vi "SetDiodeTemp.vi"() -> ()   [LabVIEW 2009]
panel:
  in  "Temp":dbl
  in  "Settling Time (s)":dbl=60.0 caption="Delay Time (s)"
  in  "+e":dbl
  in  "-e":dbl
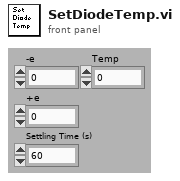
[diagram p1: front panel]
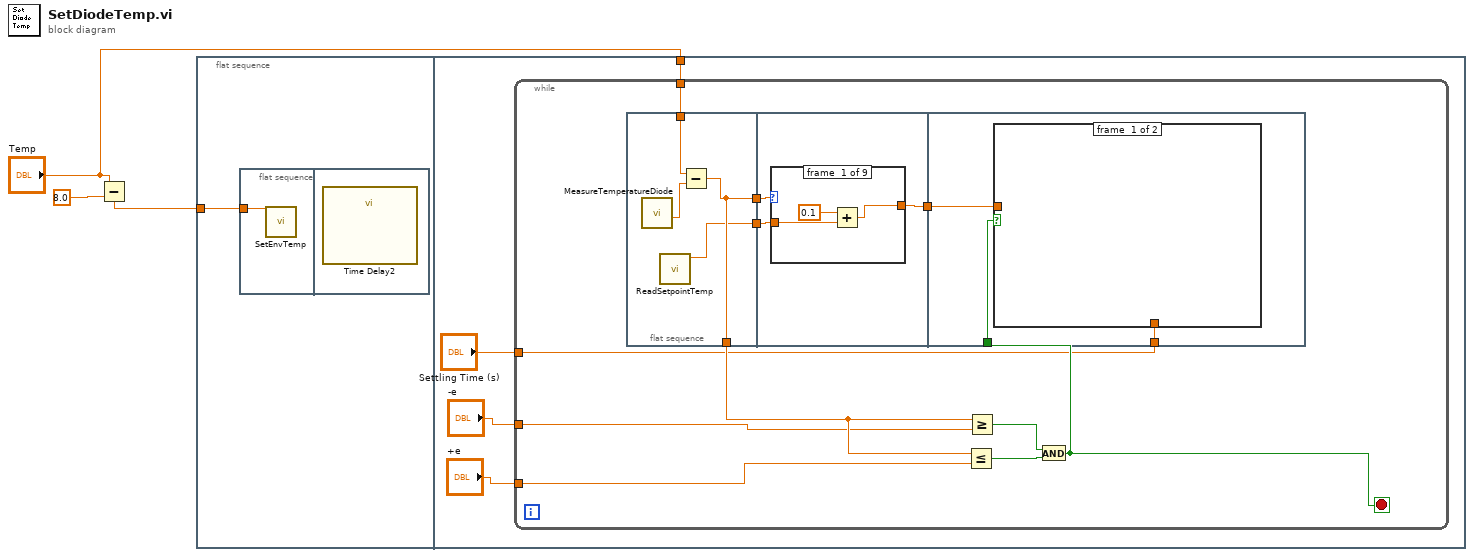
[diagram p0: block diagram]
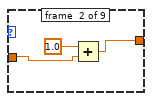
[diagram p2: hidden frame]
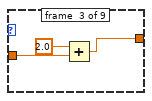
[diagram p3: hidden frame]
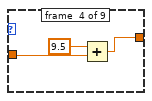
[diagram p4: hidden frame]
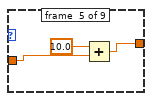
[diagram p5: hidden frame]
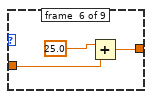
[diagram p6: hidden frame]
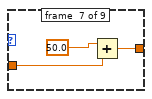
[diagram p7: hidden frame]
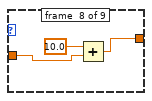
[diagram p8: hidden frame]
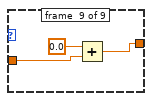
[diagram p9: hidden frame]
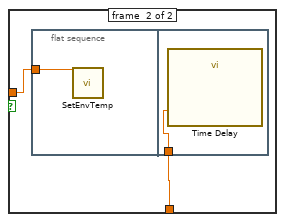
[diagram p10: hidden frame]
diagram:
  n1 = Subtract(x="Temp", y=8.0) -> (x-y=w2:dbl)
  n2 = flat-sequence {
    tunnel: w2 -> [w4]
    tunnel: "Temp" -> [w6]
    frame #0 {
      n3 = flat-sequence {
        tunnel: w4 -> [w5]
        frame #0 {
          n4 = call "SetEnvTemp.vi"("New temperature"=w5) -> ()  [unwired: 10 in, 1 out]
        }
        frame #1 {
          n5 = call "Time Delay2"() -> ()  [unwired: 11 in, 1 out]
        }
      }
    }
    frame #1 {
      n6 = while {
        tunnel: "-e" -> [w13]
        tunnel: "+e" -> [w12]
        tunnel: "Settling Time (s)" -> [w11]
        tunnel: w6 -> [w10]
        stop <- w14 stop-if-true
        n7 = flat-sequence {
          tunnel: [w22] -> w20
          tunnel: [w23] -> w18
          tunnel: [w23] -> w17
          tunnel: w10 -> [w21]
          tunnel: w20 -> [w27]
          tunnel: [w26] -> w19
          tunnel: w18 -> [w25]
          tunnel: w19 -> [w57]
          tunnel: w14 -> [w56]
          tunnel: w11 -> [w55]
          frame #0 {
            n8 = call "MeasureTemperatureDiode.vi"() -> ("Celcius"=w24:dbl)  [unwired: 8 in, 3 out]
            n9 = call "ReadSetpointTemp.vi"() -> ("Probe 1 temperature"=w22:dbl)  [unwired: 10 in, 1 out]
            n10 = Subtract(x=w21, y=w24) -> (x-y=w23:dbl)
          }
          frame #1 {
            n11 = case shown="5..10" w25 {
              tunnel: w27 -> [w30 w31 w36 w38 w41 w43 w46 w50 w53]
              tunnel: [w28 w32 w34 w37 w40 w44 w47 w49 w52] -> w26
              frame #0 {
                n12 = Add(x=0.1, y=w30) -> (x+y=w28:dbl)
              }
              frame #1 {
                n13 = Add(x=1.0, y=w31) -> (x+y=w32:dbl)
              }
              frame #2 {
                n14 = Add(x=2.0, y=w36) -> (x+y=w34:dbl)
              }
              frame #3 {
                n15 = Add(x=9.5, y=w38) -> (x+y=w37:dbl)
              }
              frame #4 {
                n16 = Add(x=10.0, y=w41) -> (x+y=w40:dbl)
              }
              frame #5 {
                n17 = Add(x=25.0, y=w43) -> (x+y=w44:dbl)
              }
              frame #6 {
                n18 = Add(x=50.0, y=w46) -> (x+y=w47:dbl)
              }
              frame #7 {
                n19 = Add(x=10.0, y=w50) -> (x+y=w49:dbl)
              }
              frame #8 {
                n20 = Add(x=0.0, y=w53) -> (x+y=w52:dbl)
              }
            }
          }
          frame #2 {
            n21 = case shown="False" w56 {
              tunnel: w57 -> [_ w59]
              tunnel: w55 -> [_ w58]
              frame #0 {
              }
              frame #1 {
                n22 = flat-sequence {
                  tunnel: w59 -> [w60]
                  tunnel: w58 -> [w61]
                  frame #0 {
                    n23 = call "SetEnvTemp.vi"("New temperature"=w60) -> ()  [unwired: 10 in, 1 out]
                  }
                  frame #1 {
                    n24 = call "Time Delay"("Delay Time (s)"=w61) -> ()  [unwired: 10 in, 1 out]
                  }
                }
              }
            }
          }
        }
        n25 = Less Or Equal?(x=w17, y=w12) -> (x <= y?=w16:bool)
        n26 = Greater Or Equal?(x=w17, y=w13) -> (x >= y?=w15:bool)
        n27 = And(x=w15, y=w16) -> (x .and. y?=w14:bool)
      }
    }
  }
